vi "Read Secret Key for License Creation.vi"(8 "error in (no error)":errorcluster, 11 "Software License Manager in":refnum<class "Software License Manager.lvclass">) -> (0 "error out":errorcluster, 2 "Secret Key for License Creation":string, 3 "Software License Manager out":refnum<class "Software License Manager.lvclass">)   [LabVIEW 2025, in "SW License Manager.lvlib" / "Software License Manager.lvclass"]
uses:
  Software License Manager.lvclass
  Software License Manager.lvclass/Software License Manager.ctl
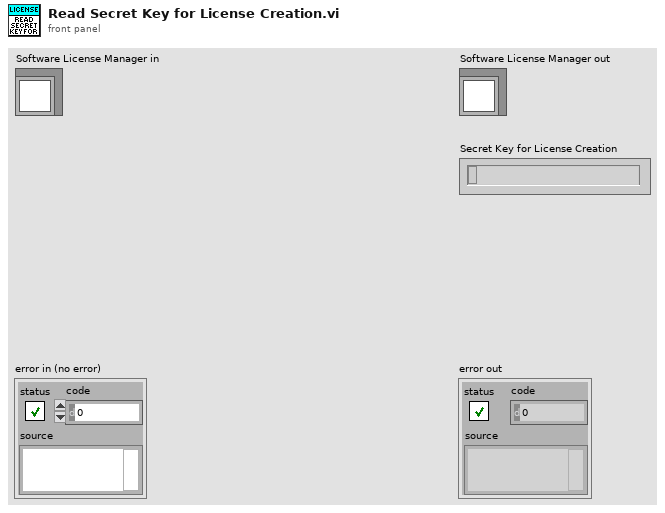
[diagram p1: front panel]
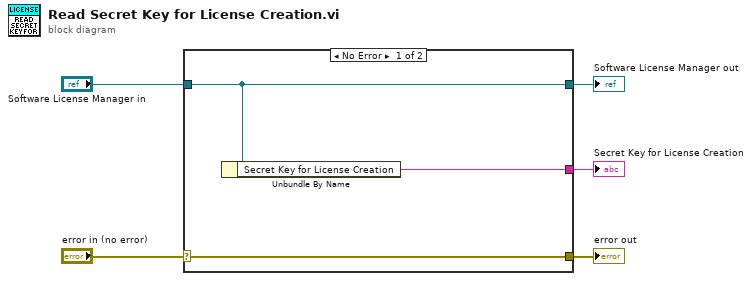
[diagram p0: block diagram]
diagram:
  n1 = case shown="No Error" "error in (no error)" {
    selector: "error in (no error)" -> [w8 w9]
    tunnel: [w8 w9] -> w4
    tunnel: [w7 w10] -> w2
    tunnel: "Software License Manager in" -> [w7 w10]
    tunnel: [w6 _] -> w1
    frame No Error {
      n2 = Unbundle By Name(w7) -> ("Secret Key for License Creation"=w6:string)
    }
    frame Error {
    }
  }
  "error out" <- w4
  "Software License Manager out" <- w2
  "Secret Key for License Creation" <- w1
